vi "Counter Get Delta T.vi"(8 "error in":errorcluster, 11 "counter session in":T1) -> (0 "error out":errorcluster, 2 "delta t [s]":dbl, 3 "counter session out":T1)   [LabVIEW 2018, in "Counter.lvlib"]
doc: "Call this to perform a single measurement of delta T interval. Counter must be first configured to the delta T mode."
uses:
  Counter.lvlib
  Counter Session.ctl
  Counter Type.ctl
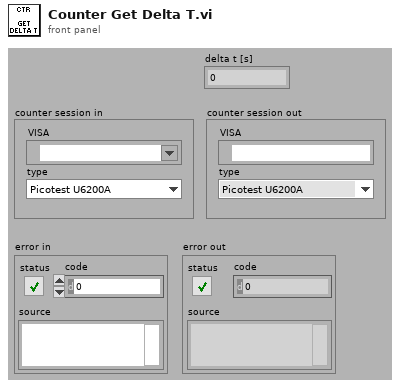
[diagram p1: front panel]
types:
  T1 = typedef "Counter.lvlib/Counter Session.ctl" = cluster{"VISA":refnum<visa-resource-name>, "type":T2}
  T2 = typedef "Counter.lvlib/Counter Type.ctl" = enum16{"Picotest U6200A", "dummy"}
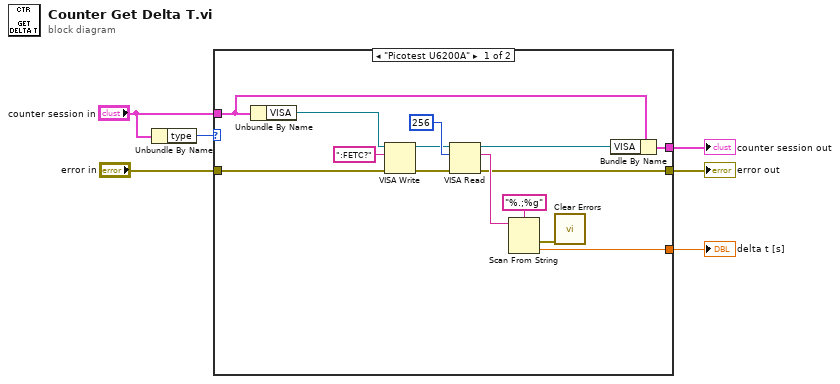
[diagram p0: block diagram]
diagram:
  n1 = Unbundle By Name("counter session in") -> ("type"=w6:T2)
  n2 = case shown="\"Picotest U6200A\"" w6 {
    tunnel: "error in" -> [w13 w22]
    tunnel: "counter session in" -> [w20 w21]
    tunnel: [w10 w22] -> w3
    tunnel: [w19 w21] -> w2
    tunnel: [w8 _] -> w1
    frame "Picotest U6200A" {
      n3 = Unbundle By Name(w20) -> ("VISA"=w12:refnum<visa-resource-name>)
      n4 = VISA Write(VISA resource name=w12, write buffer=":FETC?", error in (no error)=w13) -> (VISA resource name out=w14:refnum<visa-resource-name>, error out=w15:errorcluster)  [unwired: 1 out]
      n5 = VISA Read(VISA resource name=w14, byte count=u32 256, error in (no error)=w15) -> (VISA resource name out=w11:refnum<visa-resource-name>, read buffer=w17:string, error out=w10:errorcluster)  [unwired: 1 out]
      n6 = Scan From String(format string="%.;%g", input string=w17) -> (error out=w7:errorcluster, output 1=w8:dbl)  [unwired: 3 in, 2 out]
      n7 = call <vilib>:"Clear Errors.vi"("error in (no error)"=w7) -> ()  [unwired: 5 in, 2 out]
      n8 = Bundle By Name(cluster=w20, "VISA"=w11) -> (w19:T1)
    }
    frame Default {
    }
  }
  "error out" <- w3
  "counter session out" <- w2
  "delta t [s]" <- w1
